vi "Sistema_3_Ejes.vi"() -> ()   [LabVIEW 2017]
uses:
  <vilib>/Motion/Express/_s/nimc.ex.write.writeSetpoint.axis.vi
  <vilib>/Motion/Express/_s/nimc.ex.read.readExecutionData.axis.vi
  <vilib>/Motion/BlockNode/FB.NIMotion.xnode
panel:
  out "result":i32=7
  out "EY":dbl(slide)=3.0 scale=0.0..10.0
  out "EX":dbl(slide)=4.0 scale=0.0..10.0
  out "YZ":cluster{dbl[], dbl[]}(graph)
  out "XZ":cluster{dbl[], dbl[]}(graph)
  out "Z":dbl(slide)=4.0 scale=0.0..10.0
  in  "Array 2":cluster{"X":dbl, "Y":dbl, "Z":dbl}[](array[cluster])=[{"X"=1.0, "Y"=0.0, "Z"=0.0}, {"X"=1.0, "Y"=1.0, "Z"=1.0}, {"X"=2.0, "Y"=1.0, "Z"=2.0}, {"X"=3.0, "Y"=0.0, "Z"=3.0}, {"X"=4.0, "Y"=3.0, "Z"=4.0}]
  in  "Velocidad":dbl=2.0 format="%#_13g"
  out "x > y?":bool=TRUE
  out "done":bool=TRUE
  in  "Posición Inicial":cluster{"X":dbl, "Y":dbl, "Z":dbl}
  out "Paso":i32=4
  in  "Stop Button":bool
  out "EY":dbl(slide)=3.0 scale=0.0..10.0
  out "EX":dbl(slide)=4.0 scale=0.0..10.0
  out "XY":cluster{dbl[], dbl[]}(graph)
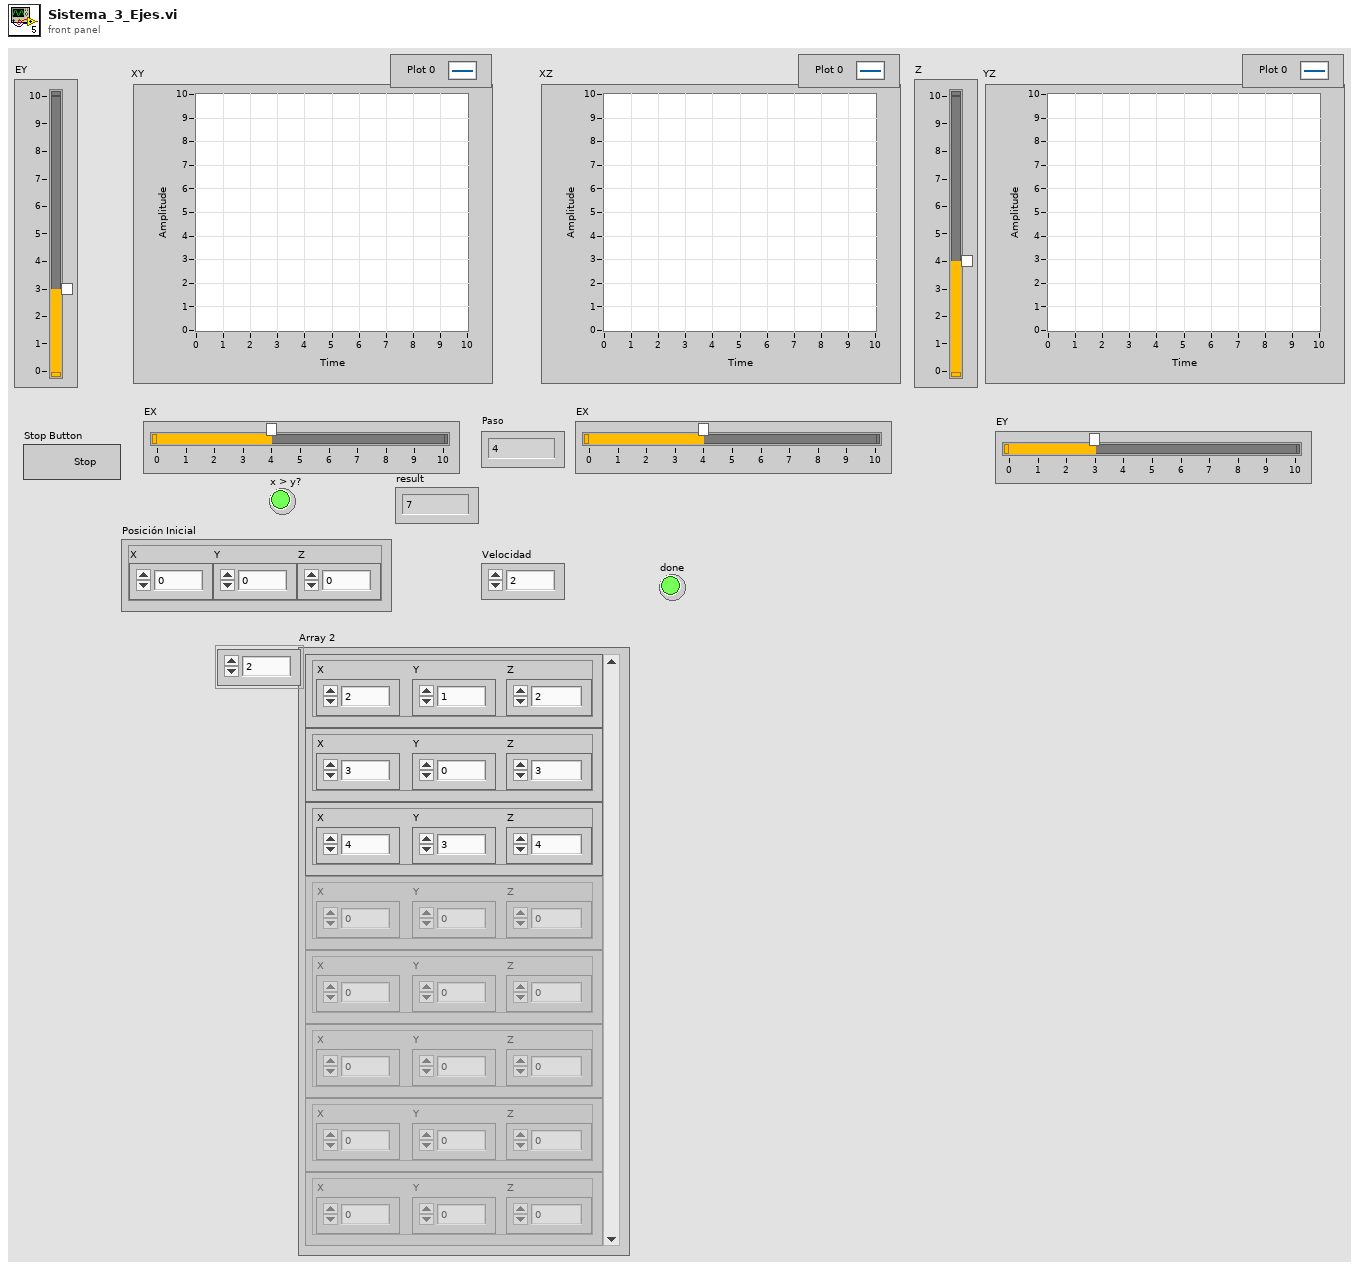
[diagram p1: front panel]
types:
  T1 = cluster{"Dif_1":dbl, "Dif_2":dbl, "Motion Resource 2":refnum<k21>, "Motion Resource 1":refnum<k21>, "Velocidad":dbl, "Posición_1":dbl, "Posición_2":dbl}
  T2 = cluster{"Motion Resource 1":refnum<k21>, "Motion Resource 2":refnum<k21>, "Motion Resource 3":refnum<k21>, "Posición_1":dbl, "Posición_2":dbl, "Posición_3":dbl, "Velocidad":dbl, "Dif_1":dbl, "Dif_2":dbl, "Dif_3":dbl}
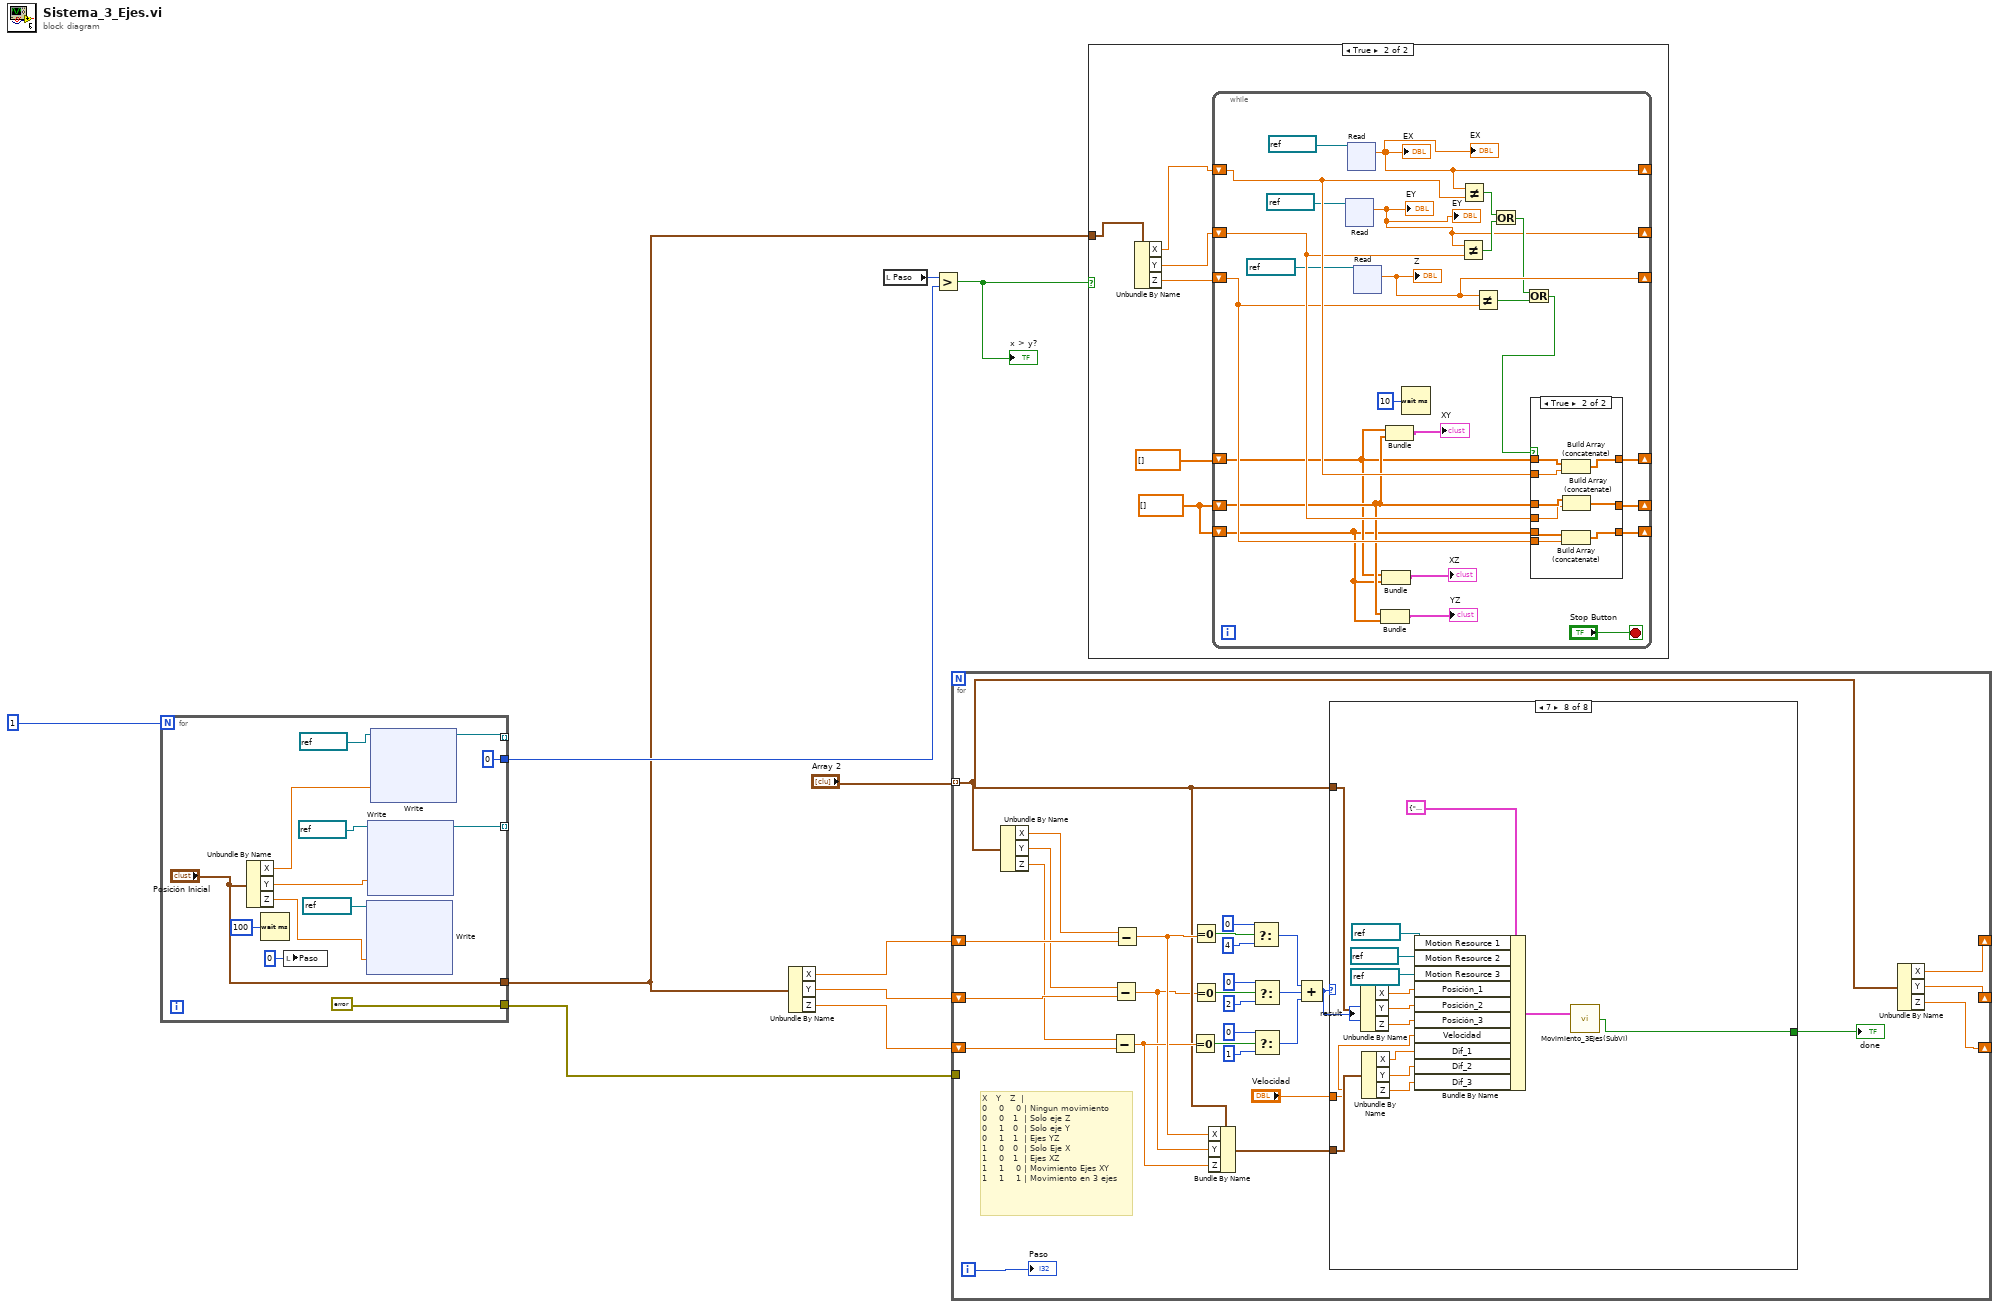
[diagram p0: block diagram]
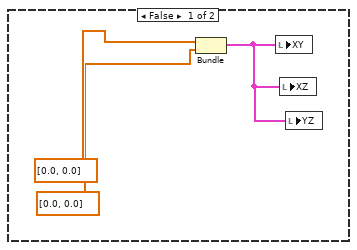
[diagram p2: hidden frame]
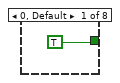
[diagram p4: hidden frame]
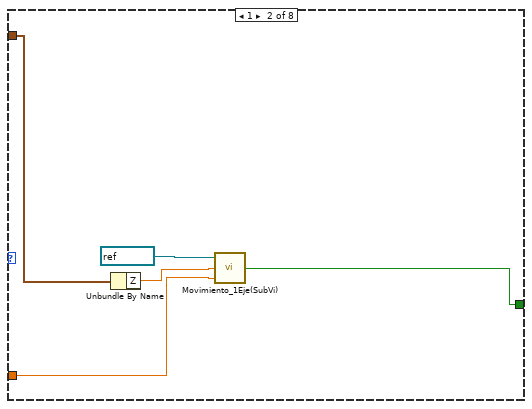
[diagram p5: hidden frame]
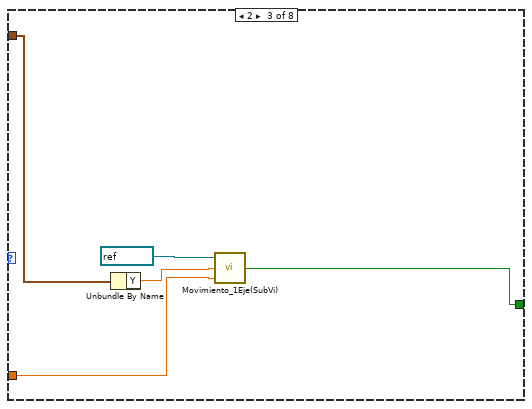
[diagram p6: hidden frame]
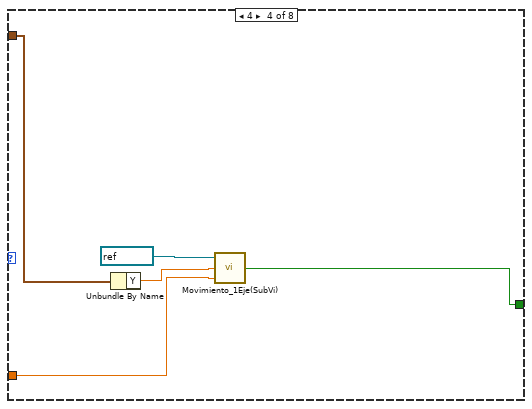
[diagram p7: hidden frame]
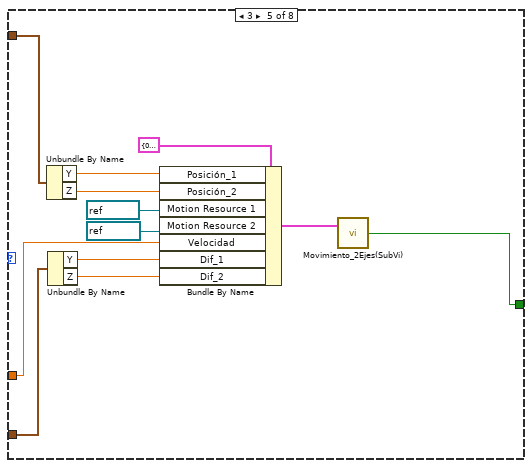
[diagram p8: hidden frame]
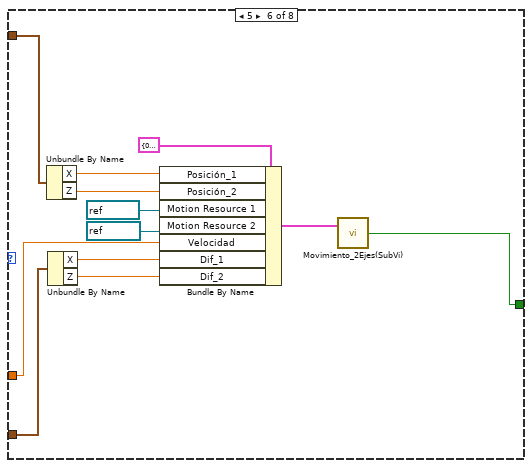
[diagram p9: hidden frame]
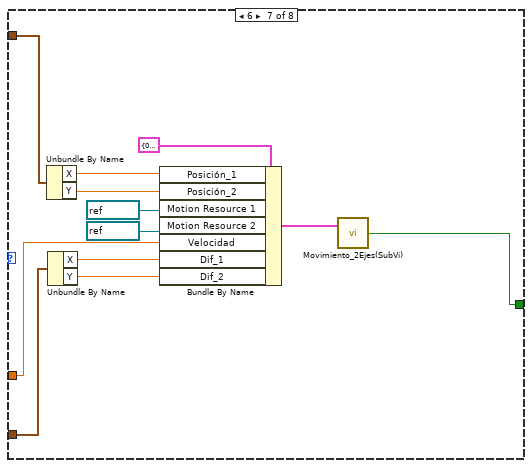
[diagram p10: hidden frame]
diagram:
  n1 = for {
    N: 1 -> [_]
    tunnel: [errorcluster {"status"=FALSE, "code"=0, "source"=""} ("error in")] -> w4
    tunnel: ["Posición Inicial"] -> w1
    tunnel: [w19] -> _ mode=indexing
    tunnel: [w18] -> _ mode=indexing
    tunnel: [0 ("y")] -> w5
    n2 = Unbundle By Name("Posición Inicial") -> ("X"=w13:dbl, "Y"=w17:dbl, "Z"=w11:dbl)
    n3 = Wait (ms)(milliseconds to wait=u32 100) -> ()  [unwired: 1 out]
    n4 = local write "Paso"(0 ("Paso")) -> ()
    n5 = xnode ("Write")("position setpoint"=w11, "resource"=refnum<k21> "EJE Z" ("Motion Resource")) -> ()  [unwired: 1 in, 2 out]
    n6 = xnode ("Write")("position setpoint"=w17, "resource"=refnum<k21> "Eje Y" ("Motion Resource")) -> ("resource out"=w19:refnum<k21>)  [unwired: 1 in, 1 out]
    n7 = xnode ("Write")("position setpoint"=w13, "resource"=refnum<k21> "Eje X" ("Motion Resource")) -> ("resource out"=w18:refnum<k21>)  [unwired: 1 in, 1 out]
  }
  n8 = Unbundle By Name(w1) -> ("X"=w9:dbl, "Y"=w8:dbl, "Z"=w2:dbl)
  n9 = local read "Paso"() -> (w7:i32)
  n10 = Greater?(x=w7, y=w5) -> (0:w6:bool)
  "x > y?" <- w6
  n11 = for {
    tunnel: "Array 2" -> [w41] mode=indexing
    tunnel: w4 -> [_]
    shift-right: [w66] -> _
    shift-left: w8 -> [w55]
    shift-right: [w67] -> _
    shift-left: w9 -> [w56]
    shift-right: [w47] -> _
    shift-left: w2 -> [w54]
    i -> [w68]
    # "X   Y   Z  |\n0    0    0 | Ningun movimiento\n0    0   1  | Solo eje Z\n0    1   0  | Solo eje Y\n0    1   1  | Ejes YZ \n1    0   0  | Solo Eje X\n1    0   1  | Ejes XZ\n1    1    0 | Movimiento Ejes XY\n1    1    1 | Movimiento en 3 ejes"
    n12 = Unbundle By Name(w41) -> ("X"=w51:dbl, "Y"=w52:dbl, "Z"=w53:dbl)
    n13 = Subtract(x=w53, y=w54) -> (x-y=w42:dbl)
    n14 = Subtract(x=w52, y=w55) -> (x-y=w40:dbl)
    n15 = Subtract(x=w51, y=w56) -> (x-y=w43:dbl)
    n16 = Equal To 0?(x=w42) -> (x = 0?=w57:bool)
    n17 = Equal To 0?(x=w43) -> (x = 0?=w65:bool)
    n18 = Equal To 0?(x=w40) -> (x = 0?=w60:bool)
    n19 = Bundle By Name(cluster=w41, "X"=w43, "Y"=w40, "Z"=w42) -> (w39:cluster{"X":dbl, "Y":dbl, "Z":dbl})
    n20 = Select(t=0, s=w65, f=4) -> (s? t:f=w49:i32)
    n21 = Select(t=0, s=w60, f=2) -> (s? t:f=w50:i32)
    n22 = Select(t=0, s=w57, f=1) -> (s? t:f=w48:i32)
    n23 = Compound Arithmetic op=ADD(w49, w50, w48) -> (w46:i32)
    "result" <- w46
    n24 = case shown="7" w46 {
      tunnel: [TRUE w70 w75 w80 w85 w97 w109 w133] -> w45
      tunnel: w41 -> [_ w73 w78 w83 w93 w105 w117 w129]
      tunnel: "Velocidad" -> [_ w71 w76 w81 w87 w99 w111 w121]
      tunnel: w39 -> [_ _ _ _ w90 w102 w114 w125]
      frame 0, Default {
      }
      frame 1 {
        n25 = Unbundle By Name(w73) -> ("Z"=w72:dbl)
        n26 = call "Movimiento_1Eje(SubVi).vi"("Velocidad"=w71, "Posición"=w72, "Motion Resource 1"=refnum<k21> "EJE Z") -> ("Done"=w70:bool)
      }
      frame 2 {
        n27 = Unbundle By Name(w78) -> ("Y"=w77:dbl)
        n28 = call "Movimiento_1Eje(SubVi).vi"("Velocidad"=w76, "Posición"=w77, "Motion Resource 1"=refnum<k21> "Eje Y") -> ("Done"=w75:bool)
      }
      frame 4 {
        n29 = Unbundle By Name(w83) -> ("Y"=w82:dbl)
        n30 = call "Movimiento_1Eje(SubVi).vi"("Velocidad"=w81, "Posición"=w82, "Motion Resource 1"=refnum<k21> "Eje X") -> ("Done"=w80:bool)
      }
      frame 3 {
        n31 = Unbundle By Name(w93) -> ("Y"=w92:dbl, "Z"=w91:dbl)
        n32 = Unbundle By Name(w90) -> ("Y"=w89:dbl, "Z"=w88:dbl)
        n33 = Bundle By Name(cluster=T1 {"Dif_1"=0.0, "Dif_2"=0.0, "Motion Resource 2"="Eje Y", "Motion Resource 1"="Eje X", "Velocidad"=0.0, "Posición_1"=0.0, "Posición_2"=0.0} ("Cluster"), "Posición_1"=w92, "Posición_2"=w91, "Motion Resource 1"=refnum<k21> "Eje Y" ("Motion Resource 2"), "Motion Resource 2"=refnum<k21> "EJE Z" ("Motion Resource 1"), "Velocidad"=w87, "Dif_1"=w89, "Dif_2"=w88) -> (w86:T1)
        n34 = call "Movimiento_2Ejes(SubVi).vi"("Cluster"=w86) -> ("Done"=w85:bool)  [unwired: 1 in]
      }
      frame 5 {
        n35 = Unbundle By Name(w105) -> ("X"=w104:dbl, "Z"=w103:dbl)
        n36 = Unbundle By Name(w102) -> ("X"=w101:dbl, "Z"=w100:dbl)
        n37 = Bundle By Name(cluster=T1 {"Dif_1"=0.0, "Dif_2"=0.0, "Motion Resource 2"="Eje Y", "Motion Resource 1"="Eje X", "Velocidad"=0.0, "Posición_1"=0.0, "Posición_2"=0.0} ("Cluster"), "Posición_1"=w104, "Posición_2"=w103, "Motion Resource 1"=refnum<k21> "Eje X" ("Motion Resource 2"), "Motion Resource 2"=refnum<k21> "EJE Z" ("Motion Resource 1"), "Velocidad"=w99, "Dif_1"=w101, "Dif_2"=w100) -> (w98:T1)
        n38 = call "Movimiento_2Ejes(SubVi).vi"("Cluster"=w98) -> ("Done"=w97:bool)  [unwired: 1 in]
      }
      frame 6 {
        n39 = Unbundle By Name(w117) -> ("X"=w116:dbl, "Y"=w115:dbl)
        n40 = Unbundle By Name(w114) -> ("X"=w113:dbl, "Y"=w112:dbl)
        n41 = Bundle By Name(cluster=T1 {"Dif_1"=0.0, "Dif_2"=0.0, "Motion Resource 2"="Eje Y", "Motion Resource 1"="Eje X", "Velocidad"=0.0, "Posición_1"=0.0, "Posición_2"=0.0} ("Cluster"), "Posición_1"=w116, "Posición_2"=w115, "Motion Resource 1"=refnum<k21> "Eje X" ("Motion Resource 2"), "Motion Resource 2"=refnum<k21> "Eje Y" ("Motion Resource 1"), "Velocidad"=w111, "Dif_1"=w113, "Dif_2"=w112) -> (w110:T1)
        n42 = call "Movimiento_2Ejes(SubVi).vi"("Cluster"=w110) -> ("Done"=w109:bool)  [unwired: 1 in]
      }
      frame 7 {
        n43 = Unbundle By Name(w129) -> ("X"=w128:dbl, "Y"=w127:dbl, "Z"=w126:dbl)
        n44 = Unbundle By Name(w125) -> ("X"=w124:dbl, "Y"=w123:dbl, "Z"=w122:dbl)
        n45 = Bundle By Name(cluster=T2 {"Motion Resource 1"="Eje X", "Motion Resource 2"="Eje Y", "Motion Resource 3"="Eje Y", "Posición_1"=0.0, "Posición_2"=0.0, "Posición_3"=0.0, "Velocidad"=0.0, "Dif_1"=0.0, "Dif_2"=0.0, "Dif_3"=0.0} ("Cluster"), "Motion Resource 1"=refnum<k21> "Eje X", "Motion Resource 2"=refnum<k21> "Eje Y", "Motion Resource 3"=refnum<k21> "EJE Z", "Posición_1"=w128, "Posición_2"=w127, "Posición_3"=w126, "Velocidad"=w121, "Dif_1"=w124, "Dif_2"=w123, "Dif_3"=w122) -> (w134:T2)
        n46 = call "Movimiento_3Ejes(SubVi).vi"("Cluster"=w134) -> ("Done"=w133:bool)  [unwired: 1 in]
      }
    }
    "done" <- w45
    n47 = Unbundle By Name(w41) -> ("X"=w67:dbl, "Y"=w66:dbl, "Z"=w47:dbl)
    "Paso" <- w68
  }
  n48 = case shown="True" w6 {
    tunnel: w1 -> [_ w142]
    frame False {
      n49 = Bundle(dbl[] [0.0, 0.0], dbl[] [0.0, 0.0]) -> (w136:cluster{dbl[], dbl[]})  [unwired: 1 in]
      n50 = local write "XY"(w136) -> ()
      n51 = local write "XZ"(w136) -> ()
      n52 = local write "YZ"(w136) -> ()
    }
    frame True {
      w143 = dbl[] []
      n53 = Unbundle By Name(w142) -> ("X"=w141:dbl, "Y"=w140:dbl, "Z"=w139:dbl)
      n54 = while {
        shift-right: [w146] -> _
        shift-left: w141 -> [w167]
        shift-right: [w145] -> _
        shift-left: w140 -> [w166]
        shift-right: [w165] -> _
        shift-left: w143 -> [w149]
        shift-right: [w164] -> _
        shift-left: dbl[] [] -> [w148]
        shift-right: [w157] -> _
        shift-left: w139 -> [w152]
        shift-right: [w153] -> _
        shift-left: w143 -> [w147]
        stop <- "Stop Button" stop-if-true
        n55 = xnode "Read"("resource"=refnum<k21> "Eje Y" ("Motion Resource")) -> ("position"=w145:dbl)  [unwired: 1 in, 6 out]
        "EY" <- w145
        "EY" <- w145
        n56 = xnode "Read"("resource"=refnum<k21> "Eje X" ("Motion Resource")) -> ("position"=w146:dbl)  [unwired: 1 in, 6 out]
        "EX" <- w146
        "EX" <- w146
        n57 = xnode "Read"("resource"=refnum<k21> "EJE Z" ("Motion Resource")) -> ("position"=w157:dbl)  [unwired: 1 in, 6 out]
        "Z" <- w157
        n58 = Bundle(w149, w147) -> (→"YZ":cluster{dbl[], dbl[]})  [unwired: 1 in]
        n59 = Bundle(w148, w147) -> (→"XZ":cluster{dbl[], dbl[]})  [unwired: 1 in]
        n60 = Bundle(w148, w149) -> (→"XY":cluster{dbl[], dbl[]})  [unwired: 1 in]
        n61 = Wait (ms)(milliseconds to wait=u32 10) -> ()  [unwired: 1 out]
        n62 = Not Equal?(x=w145, y=w166) -> (x != y?=w168:bool)
        n63 = Not Equal?(x=w146, y=w167) -> (x != y?=w169:bool)
        n64 = Not Equal?(x=w157, y=w152) -> (x != y?=w156:bool)
        n65 = Or(x=w169, y=w168) -> (x .or. y?=w155:bool)
        n66 = Or(x=w155, y=w156) -> (x .or. y?=w154:bool)
        n67 = case shown="True" w154 {
          tunnel: w148 -> [w181 w190]
          tunnel: w149 -> [w180 w187]
          tunnel: w167 -> [_ w189]
          tunnel: w166 -> [_ w186]
          tunnel: [w180 w185] -> w165
          tunnel: [w181 w188] -> w164
          tunnel: w147 -> [w179 w184]
          tunnel: [w179 w182] -> w153
          tunnel: w152 -> [_ w183]
          frame False {
          }
          frame True {
            n68 = Build Array (concatenate)(w190, w189) -> (w188:dbl[])
            n69 = Build Array (concatenate)(w184, w183) -> (w182:dbl[])
            n70 = Build Array (concatenate)(w187, w186) -> (w185:dbl[])
          }
        }
      }
    }
  }
